vi "To Pretty String (Null).vi"(7 "enable LabVIEW extensions? (T)":bool=TRUE, 8 "error in (no error)":errorcluster, 10 "indent":i32, 11 "JSON Datatype in":refnum<class "JSON Value.lvclass">) -> (0 "error out":errorcluster, 3 "String":string)   [LabVIEW 2016, in "JSON Value.lvclass"]
doc: "Flattens the given JSON data to a string."
uses:
  JSON Value.lvclass
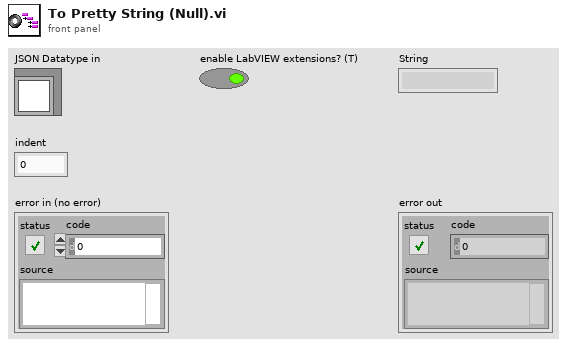
[diagram p1: front panel]
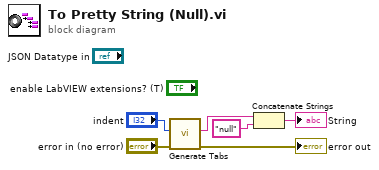
[diagram p0: block diagram]
diagram:
  n1 = call "Generate Tabs.vi"("error in (no error)"="error in (no error)", "indent"="indent") -> ("error out"=→"error out":errorcluster, "Tabs"=w5:string)  [unwired: 8 in]
  n2 = Concatenate Strings(w5, "null" ("String")) -> (→"String":string)
